vi "GetHeightAdj.vi"(1 "appended path":path) -> (0 "Numeric":dbl)   [LabVIEW 2013, in "main.lvlib"]
uses:
  main.lvlib
  <userlib>/_OpenG.lib/file/file.llb/File Exists - Scalar__ogtk.vi
  <vilib>/Utility/file.llb/Read From Spreadsheet File (DBL).vi
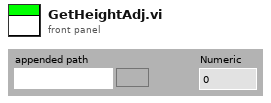
[diagram p1: front panel]
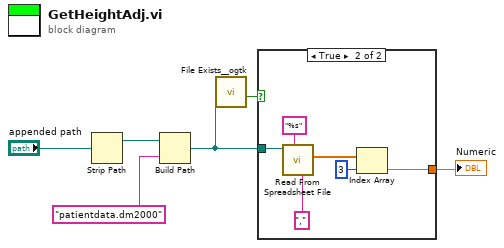
[diagram p0: block diagram]
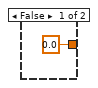
[diagram p2: hidden frame]
diagram:
  n1 = Strip Path(path="appended path") -> (stripped path=w5:path)  [unwired: 1 out]
  n2 = Build Path(base path=w5, name or relative path="patientdata.dm2000") -> (appended path=w2:path)
  n3 = call-poly <userlib>:"File Exists__ogtk.vi"("file path"=w2) -> ("exists"=w3:bool)  [unwired: 6 in, 1 out]
  n4 = case shown="True" w3 {
    tunnel: w2 -> [_ w9]
    tunnel: [0.0 w8] -> w1
    frame False {
    }
    frame True {
      n5 = call-poly <vilib>:"Read From Spreadsheet File.vi"("delimiter (\\t)"="," ("delimiter (\\t)"), "format (%.3f)"="%s", "file path (dialog if empty)"=w9) -> ("first row"=w10:dbl[])  [unwired: 4 in, 4 out]
      n6 = Index Array(array=w10, index=3) -> (element=w8:dbl)
    }
  }
  "Numeric" <- w1
